vi "Send Write Settings to File Sync.vi"(7 "Message Priority (Normal)":T2=enum."Normal", 8 "error in (no error)":errorcluster, 9 "timeout in ms (1000)":i32=1000, 10 "file refnum":T1, 11 "Message Enqueuer in":refnum<class "Message Enqueuer.lvclass">) -> (0 "error out":errorcluster, 1 "timed out?":bool, 2 "file ref":T1, 3 "Message Enqueuer out":refnum<class "Message Enqueuer.lvclass">)   [LabVIEW 2014, in "Camera Actor.lvlib" / "Write Settings to Ini File.lvclass"]
uses:
  Write Settings to Ini File.lvclass
  <vilib>/ActorFramework/Message Enqueuer/Message Priority.ctl
  <vilib>/ActorFramework/Message Enqueuer/Message Enqueuer.lvclass
  <vilib>/Utility/config.llb/Config Data RefNum.ctl
  Write Settings to Ini File.lvclass/Write Settings to Ini File.ctl
  <vilib>/ActorFramework/Reply Msg/Reply Msg.lvclass/Reply Msg.ctl
  <vilib>/ActorFramework/Message Enqueuer/Message Enqueuer.lvclass/Message Enqueuer.ctl
  <vilib>/ActorFramework/Message Enqueuer/Enqueue.vi
  <vilib>/ActorFramework/Message Priority Queue/Priority Enqueue.vi
  <vilib>/ActorFramework/Reply Msg/Reply Msg.lvclass
  <vilib>/Utility/config.llb/NI_LVConfig.lvlib
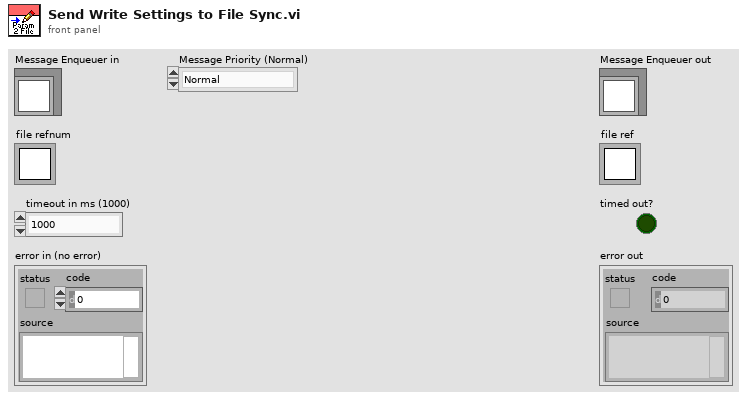
[diagram p1: front panel]
types:
  T1 = typedef "NI_LVConfig.lvlib/Config Data RefNum.ctl" = refnum<k1>
  T2 = typedef "Actor Framework.lvlib/Message Enqueuer.lvclass/Message Priority.ctl" = enum16{"Low", "Normal", "High"}
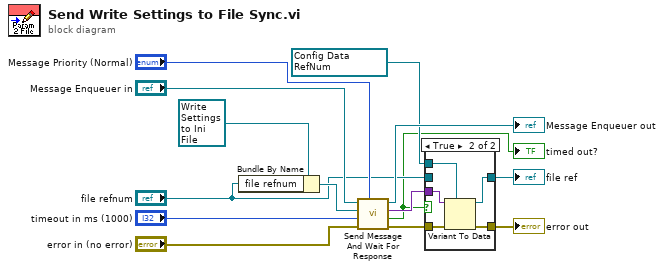
[diagram p0: block diagram]
diagram:
  w6 = T1 refnum items=["config data"] ("file refnum")
  n1 = Bundle By Name(cluster=refnum<class "Write Settings to Ini File.lvclass"> refnum ("IMAQdx Actor.lvlib:Write Settings to Ini File.lvclass"), "file refnum"="file refnum") -> (w8:refnum<class "Write Settings to Ini File.lvclass">)
  n2 = call <vilib>:"Send Message And Wait For Response.vi"("Message Priority (Normal)"="Message Priority (Normal)", "error in (no error)"="error in (no error)", "timeout in ms (-1)"="timeout in ms (1000)", "Original Message"=w8, "Message Enqueuer in"="Message Enqueuer in") -> ("error out"=w4:errorcluster, "timed out?"=w1:bool, "Reply"=w7:variant, "Message Enqueuer out"=→"Message Enqueuer out":refnum<class "Message Enqueuer.lvclass">)  [unwired: 3 in]
  "timed out?" <- w1
  n3 = case shown="True" w1 {
    tunnel: w7 -> [_ w21]
    tunnel: w6 -> [_ w20]
    tunnel: [w16 w19] -> w5
    tunnel: w4 -> [w15 w18]
    tunnel: [w15 w17] -> w3
    tunnel: "file refnum" -> [w16 _]
    frame False {
    }
    frame True {
      n4 = Variant To Data(error in=w18, type=w20, Variant=w21) -> (data=w19:T1, error out=w17:errorcluster)
    }
  }
  "error out" <- w3
  "file ref" <- w5
